vi "Post-Install Custom Action.vi"(10 "Variant":variant) -> (0 "error out":errorcluster)   [LabVIEW 2017]
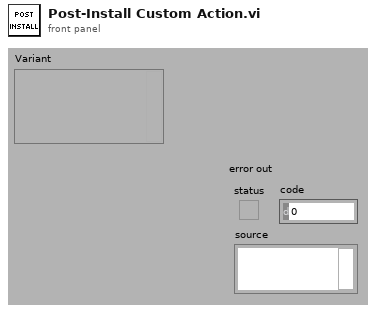
[diagram p1: front panel]
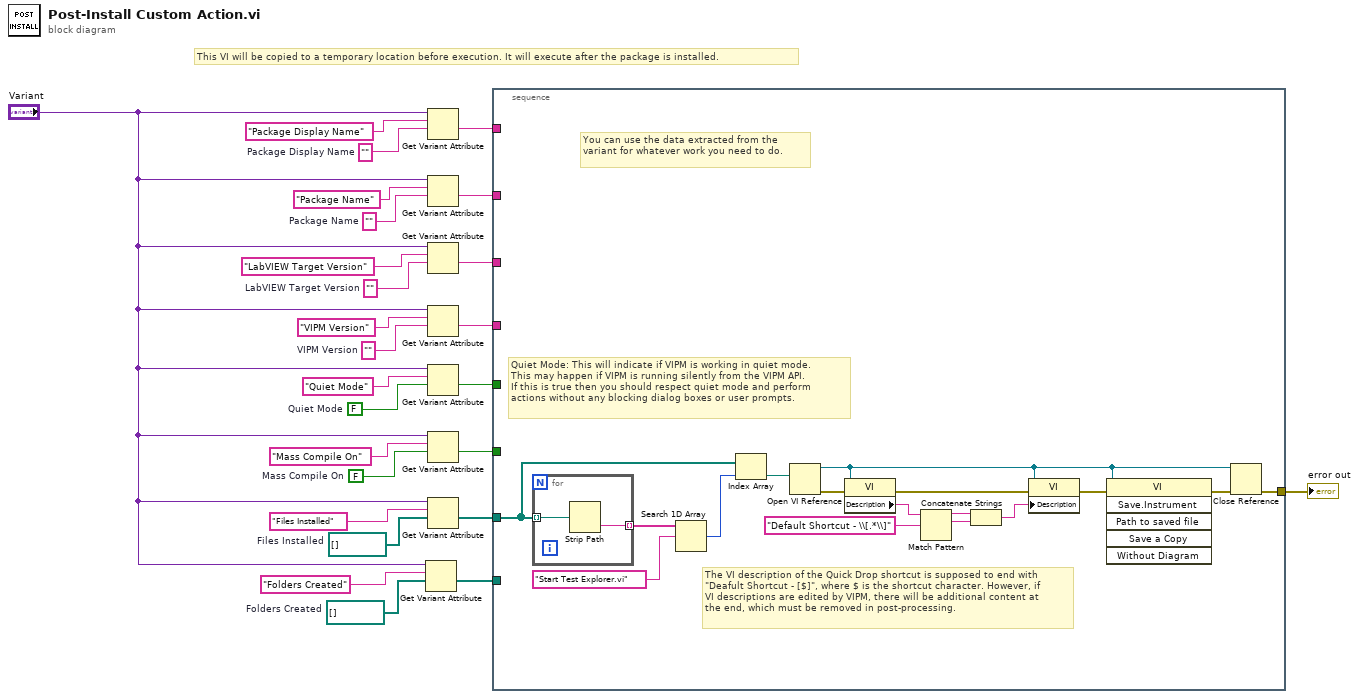
[diagram p0: block diagram]
diagram:
  w2 = path[] []  # Folders Created
  w3 = path[] []  # Files Installed
  w9 = FALSE  # Mass Compile On
  w10 = ""  # Package Display Name
  w17 = FALSE  # Quiet Mode
  w20 = ""  # VIPM Version
  w22 = ""  # LabVIEW Target Version
  w24 = ""  # Package Name
  # "This VI will be copied to a temporary location before execution. It will execute after the package is installed."
  n1 = Get Variant Attribute(Variant="Variant", name="Folders Created", default value (empty Variant)=w2) -> (value=w7:path[])  [unwired: 1 in, 3 out]
  n2 = Get Variant Attribute(Variant="Variant", name="Package Display Name", default value (empty Variant)=w10) -> (value=w16:string)  [unwired: 1 in, 3 out]
  n3 = Get Variant Attribute(Variant="Variant", name="Package Name", default value (empty Variant)=w24) -> (value=w15:string)  [unwired: 1 in, 3 out]
  n4 = Get Variant Attribute(Variant="Variant", name="LabVIEW Target Version", default value (empty Variant)=w22) -> (value=w14:string)  [unwired: 1 in, 3 out]
  n5 = Get Variant Attribute(Variant="Variant", name="VIPM Version", default value (empty Variant)=w20) -> (value=w13:string)  [unwired: 1 in, 3 out]
  n6 = Get Variant Attribute(Variant="Variant", name="Quiet Mode", default value (empty Variant)=w17) -> (value=w12:bool)  [unwired: 1 in, 3 out]
  n7 = Get Variant Attribute(Variant="Variant", name="Mass Compile On", default value (empty Variant)=w9) -> (value=w11:bool)  [unwired: 1 in, 3 out]
  n8 = Get Variant Attribute(Variant="Variant", name="Files Installed", default value (empty Variant)=w3) -> (value=w6:path[])  [unwired: 1 in, 3 out]
  n9 = stacked-sequence {
    tunnel: w16 -> [_]
    tunnel: w15 -> [_]
    tunnel: w14 -> [_]
    tunnel: w13 -> [_]
    tunnel: w12 -> [_]
    tunnel: w11 -> [_]
    tunnel: w6 -> [w40]
    tunnel: w7 -> [_]
    tunnel: [w33] -> w1
    frame #0 {
      # "The VI description of the Quick Drop shortcut is supposed to end with\n\"Deafult Shortcut - [$]\", where $ is the shortcut character. However, if\nVI descriptions are edited by VIPM, there will be additional content at\nthe end, which must be removed in post-processing."
      # "Quiet Mode: This will indicate if VIPM is working in quiet mode.\nThis may happen if VIPM is running silently from the VIPM API.\nIf this is true then you should respect quiet mode and perform\nactions without any blocking dialog boxes or user prompts."
      # "You can use the data extracted from the variant for whatever work you need to do."
      n10 = for {
        tunnel: w40 -> [w44] mode=indexing
        tunnel: [w43] -> w42 mode=indexing
        n11 = Strip Path(path=w44) -> (name=w43:string)  [unwired: 1 out]
      }
      n12 = Search 1D Array(1D array=w42, element="Start Test Explorer.vi") -> (index of element=w39:i32)  [unwired: 1 in]
      n13 = Index Array(array=w40, index=w39) -> (element=w32:path)
      n14 = Open VI Reference(vi path=w32) -> (vi reference=w34:refnum<vi>, error out=w38:errorcluster)  [unwired: 5 in]
      n15 = property class="VI"(reference=w34, error in=w38) -> (error out=w37:errorcluster, "Description"=w30:string)  [unwired: 1 out]
      n16 = Match Pattern(string=w30, regular expression="Default Shortcut - \\[.*\\]") -> (before substring=w29:string, match substring=w28:string)  [unwired: 1 in, 2 out]
      n17 = Concatenate Strings(w29, w28) -> (w27:string)
      n18 = property class="VI"(reference=w34, error in=w37, "Description"=w27) -> (error out=w36:errorcluster)  [unwired: 1 out]
      n19 = invoke class="VI" method="Save.Instrument"(reference=w34, error in=w36) -> (error out=w35:errorcluster)  [unwired: 4 in, 5 out]
      n20 = Close Reference(reference=w34, error in (no error)=w35) -> (error out=w33:errorcluster)
    }
  }
  "error out" <- w1
